vi "BRig_RT__Case_Exp__State_start__sendExpData_uploadData.vi"(8 "input_error":errorcluster, 11 "input_hSession":T1) -> ()   [LabVIEW 2014]
uses:
  <vilib>/WebDAVClient/Advanced/SessionHandle.ctl
  <vilib>/WebDAVClient/Advanced/Put File.vi
  <vilib>/WebDAVClient/NI_WebDAV.lvlib
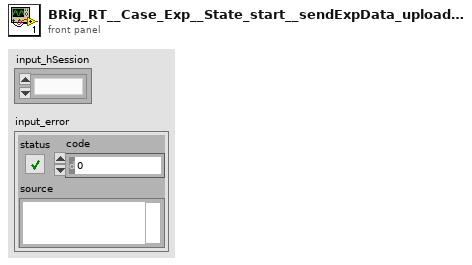
[diagram p1: front panel]
types:
  T1 = typedef "NI_WebDAV.lvlib/SessionHandle.ctl" = refnum<k1>
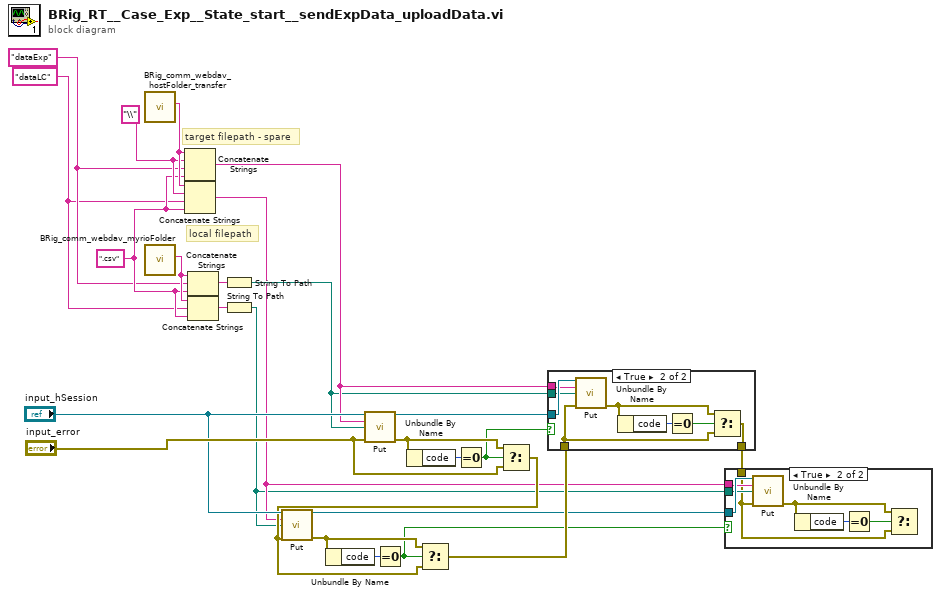
[diagram p0: block diagram]
diagram:
  w21 = "\\" ("string")
  w18 = "dataLC" ("input_filename")
  w19 = "dataExp" ("input_filename")
  w20 = ".csv" ("string")
  # "target filepath - spare"
  # "local filepath"
  n1 = call "BRig_comm_webdav_hostFolder_transfer.vi"() -> ("output_HostFolder"=w22:string)  [unwired: 11 in]
  n2 = call "BRig_comm_webdav_myrioFolder.vi"() -> ("output_myrioFolder"=w23:string)  [unwired: 11 in]
  n3 = Concatenate Strings(w22, w21, w19, w20) -> (w7:string)
  n4 = Concatenate Strings(w22, w21, w18, w20) -> (w4:string)
  n5 = Concatenate Strings(w23, w19, w20) -> (w25:string)
  n6 = Concatenate Strings(w23, w18, w20) -> (w24:string)
  n7 = String To Path(string=w25) -> (path=w6:path)
  n8 = String To Path(string=w24) -> (path=w3:path)
  n9 = call-poly <vilib>:"Put.vi"("session handle"="input_hSession", "relative uri"=w7, "local file path"=w6, "error in (no error)"="input_error") -> ("session handle out"=w8:T1, "error out"=w16:errorcluster)  [unwired: 9 in, 1 out]
  n10 = Unbundle By Name(w16) -> ("code"=w17:i32)
  n11 = Equal To 0?(x=w17) -> (x = 0?=w10:bool)
  n12 = Select(t=w16, s=w10, f="input_error") -> (s? t:f=w11:errorcluster)
  n13 = call-poly <vilib>:"Put.vi"("session handle"="input_hSession", "relative uri"=w4, "local file path"=w3, "error in (no error)"=w11) -> ("session handle out"=w5:T1, "error out"=w12:errorcluster)  [unwired: 9 in, 1 out]
  n14 = Unbundle By Name(w12) -> ("code"=w13:i32)
  n15 = Equal To 0?(x=w13) -> (x = 0?=w2:bool)
  n16 = Select(t=w12, s=w2, f=w11) -> (s? t:f=w9:errorcluster)
  n17 = case shown="True" w10 {
    tunnel: w9 -> [w26 w31]
    tunnel: w8 -> [_ w30]
    tunnel: w7 -> [_ w29]
    tunnel: w6 -> [_ w28]
    tunnel: [w26 w27] -> w1
    frame False {
    }
    frame True {
      n18 = call-poly <vilib>:"Put.vi"("session handle"=w30, "relative uri"=w29, "local file path"=w28, "error in (no error)"=w31) -> ("error out"=w33:errorcluster)  [unwired: 9 in, 2 out]
      n19 = Unbundle By Name(w33) -> ("code"=w32:i32)
      n20 = Equal To 0?(x=w32) -> (x = 0?=w34:bool)
      n21 = Select(t=w33, s=w34, f=w31) -> (s? t:f=w27:errorcluster)
    }
  }
  n22 = case shown="True" w2 {
    tunnel: w5 -> [_ w38]
    tunnel: w4 -> [_ w37]
    tunnel: w3 -> [_ w36]
    tunnel: w1 -> [_ w35]
    frame False {
    }
    frame True {
      n23 = call-poly <vilib>:"Put.vi"("session handle"=w38, "relative uri"=w37, "local file path"=w36, "error in (no error)"=w35) -> ("error out"=w40:errorcluster)  [unwired: 9 in, 2 out]
      n24 = Unbundle By Name(w40) -> ("code"=w39:i32)
      n25 = Equal To 0?(x=w39) -> (x = 0?=w41:bool)
      n26 = Select(t=w40, s=w41, f=w35) -> ()  [unwired: 1 out]
    }
  }
